vi "PDFF_Control_X.vi"(0 "Ts":dbl=0.001 format="%#_13g", 1 "Kp":dbl=460.0 format="%#_13g", 2 "Kd":dbl=4.0 format="%#_13g", 3 "FF":dbl=5975.0 format="%#_13g", 5 "e(k)":dbl, 6 "r(k)":dbl) -> (4 "u(k)":dbl, 7 "e(k)":dbl)   [LabVIEW 2015]
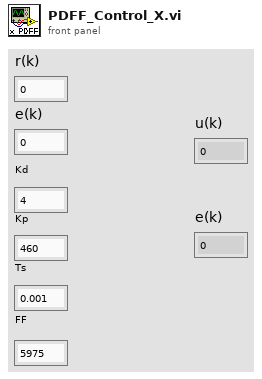
[diagram p1: front panel]
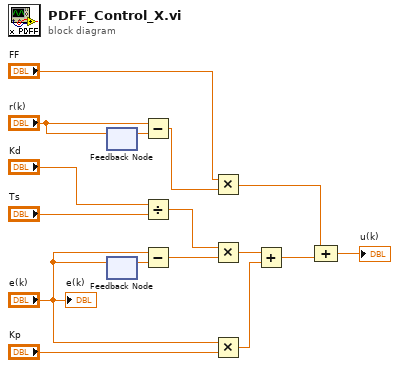
[diagram p0: block diagram]
diagram:
  n1 = feedback #1() -> (w7:dbl)  [unwired: 1 in]
  n2 = feedback-in #1("r(k)") -> ()
  n3 = feedback #2() -> (w16:dbl)  [unwired: 1 in]
  n4 = feedback-in #2("e(k)") -> ()
  n5 = Subtract(x="r(k)", y=w7) -> (x-y=w3:dbl)
  n6 = Divide(x="Kd", y="Ts") -> (x/y=w11:dbl)
  n7 = Subtract(x="e(k)", y=w16) -> (x-y=w15:dbl)
  n8 = Multiply(x="FF", y=w3) -> (x*y=w8:dbl)
  n9 = Multiply(x=w11, y=w15) -> (x*y=w14:dbl)
  n10 = Multiply(x="e(k)", y="Kp") -> (x*y=w13:dbl)
  n11 = Add(x=w14, y=w13) -> (x+y=w5:dbl)
  n12 = Compound Arithmetic op=ADD(w8, w5) -> (→"u(k)":dbl)
  "e(k)" <- "e(k)"
